vi "Servo Drive Test.vi"() -> ()   [LabVIEW 2020]
uses:
  <vilib>/MakerHub/LINX/LMH-LINX.lvlib
  LINX-PCA9685 PWM/LINX-PCA9685 PWM.lvclass
  LINX I2C/LINX I2C.lvclass
  <vilib>/MakerHub/LINX/Public/Utilities/Open Local.vi
panel:
  in  "PWM1":dbl(slide) scale=-100.0..100.0
  in  "PWM0":dbl(slide) scale=-100.0..100.0
  out "New Frequency (Hz)":dbl
  out "Initial Frequency (Hz)":dbl
  in  "stop":bool
  out "Error Out":errorcluster
  # "A simple example of driving two servo motors with a Raspberry Pi using the PCA9685 PWM driver chip.\n\nThe board provides 16 PWM channels for driving LEDs or Servos."
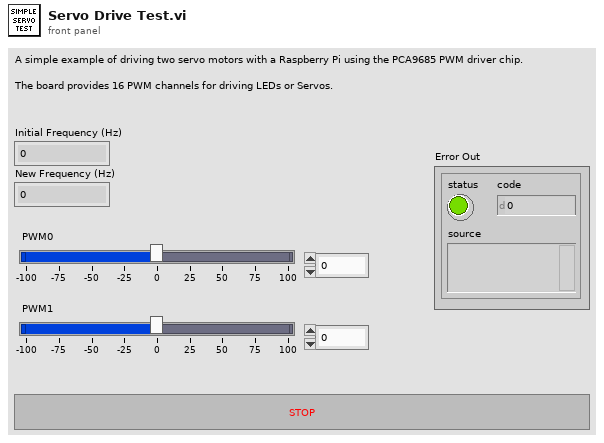
[diagram p1: front panel]
types:
  T1 = typedef "LMH-LINX.lvlib/LINX Ref.ctl" = cluster{"IO":T2, "Interface":T3, "LINX Device Config":T4}
  T2 = typedef "LMH-LINX.lvlib/Platform.ctl" = enum16{"Remote", "Local"}
  T3 = typedef "LMH-LINX.lvlib/Interface.ctl" = enum16{"Serial", "TCP"}
  T4 = typedef "LMH-LINX.lvlib/Device.lvlib/LINX Device Config.ctl" = cluster{"Interface":T3, "COM Port":refnum<visa-resource-name>, "TCP Configuration":T5, "Device Family":u8, "Device ID":u8, "Device Name":string, "TCP Ref":refnum<k5>, "Channels":T6}
  T5 = typedef "LMH-LINX.lvlib/Device.lvlib/TCP Config.ctl" = cluster{"IP Address":string, "Port":u16}
  T6 = typedef "LMH-LINX.lvlib/Channels.ctl" = cluster{"DI":u8[], "DO":u8[], "AI":u8[], "AO":u8[], "PWM":u8[], "QE":u8[], "UART":u8[], "I2C 2":u8[], "SPI":u8[], "CAN":u8[], "Servo":u8[], "AI Ref (V)":dbl, "AI Resolution (Bits)":u8, "AO Ref (V)":dbl, "AO Resolution (Bits)":u8}
  T7 = enum16{"LED/PWM00", "LED/PWM01", "LED/PWM02", "LED/PWM03", "LED/PWM04", "LED/PWM05", "LED/PWM06", "LED/PWM07", "LED/PWM08", "LED/PWM09", "LED/PWM10", "LED/PWM11", "LED/PWM12", "LED/PWM13", "LED/PWM14", "LED/PWM15"}[]
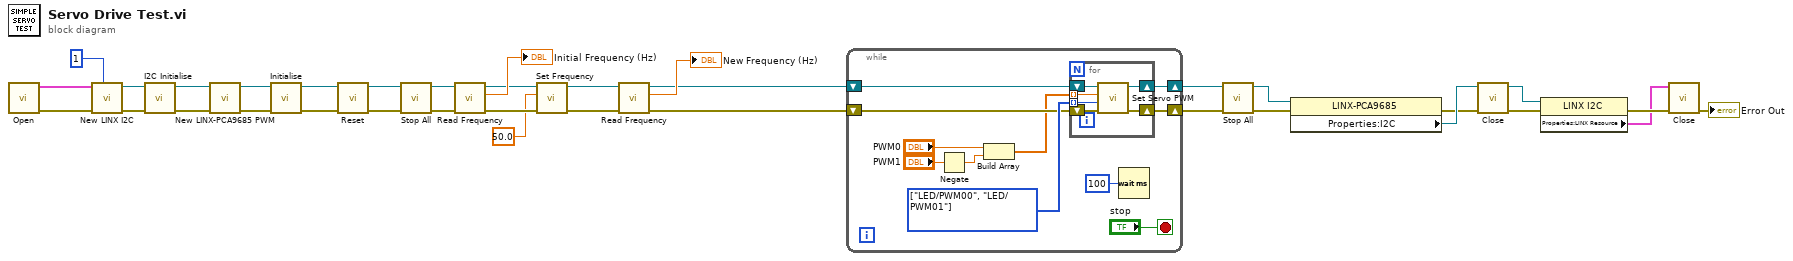
[diagram p0: block diagram]
diagram:
  n1 = call-poly <vilib>:"Open.vi"() -> ("Error Out"=w14:errorcluster, "LINX Resource"=w15:T1)  [unwired: 9 in, 1 out]
  n2 = call "New LINX I2C.vi"("LINX I2C Channel"=u8 1 ("I2C Channel"), "error in (no error)"=w14, "LINX Resource"=w15) -> ("error out"=w12:errorcluster, "LINX I2C out"=w11:refnum<class "LINX I2C.lvclass">)  [unwired: 7 in]
  n3 = call-dynamic "I2C Initialise.vi"("error in (no error)"=w12, "LINX I2C in"=w11) -> ("error out"=w4:errorcluster, "LINX I2C out"=w3:refnum<class "LINX I2C.lvclass">)  [unwired: 8 in]
  n4 = call "New LINX-PCA9685 PWM.vi"("error in (no error)"=w4, "I2C"=w3) -> ("error out"=w2:errorcluster, "LINX-PCA9865 PWM out"=w1:refnum<class "LINX-PCA9685 PWM.lvclass">)  [unwired: 8 in]
  n5 = call-dynamic "Initialise.vi"("error in (no error)"=w2, "PWM in"=w1) -> ("error out"=w19:errorcluster, "PWM out"=w20:refnum<class "LINX-PCA9685 PWM.lvclass">)  [unwired: 8 in]
  n6 = call-dynamic "Reset.vi"("error in (no error)"=w19, "PWM in"=w20) -> ("error out"=w18:errorcluster, "PWM out"=w17:refnum<class "LINX-PCA9685 PWM.lvclass">)  [unwired: 8 in]
  n7 = call-dynamic "Stop All.vi"("error in (no error)"=w18, "LINX-PCA9865 PWM in"=w17) -> ("error out"=w27:errorcluster, "LINX-PCA9865 PWM out"=w28:refnum<class "LINX-PCA9685 PWM.lvclass">)  [unwired: 8 in]
  n8 = call-dynamic "Read Frequency.vi"("error in (no error)"=w27, "PWM in"=w28) -> ("error out"=w33:errorcluster, "Frequency (Hz)"=→"Initial Frequency (Hz)":dbl, "PWM out"=w32:refnum<class "LINX-PCA9685 PWM.lvclass">)  [unwired: 7 in]
  n9 = call-dynamic "Set Frequency.vi"("error in (no error)"=w33, "Frequency (1000Hz)"=50.0, "PWM in"=w32) -> ("error out"=w31:errorcluster, "PWM out"=w30:refnum<class "LINX-PCA9685 PWM.lvclass">)  [unwired: 7 in]
  n10 = call-dynamic "Read Frequency.vi"("error in (no error)"=w31, "PWM in"=w30) -> ("error out"=w24:errorcluster, "Frequency (Hz)"=→"New Frequency (Hz)":dbl, "PWM out"=w25:refnum<class "LINX-PCA9685 PWM.lvclass">)  [unwired: 7 in]
  n11 = while {
    shift-right: [w43] -> w26
    shift-left: w24 -> [w40]
    shift-right: [w42] -> w23
    shift-left: w25 -> [w44]
    stop <- "stop" stop-if-true
    w41 = T7 [enum."LED/PWM00", enum."LED/PWM01"] items=["LED/PWM00", "LED/PWM01", "LED/PWM02", "LED/PWM03", "LED/PWM04", "LED/PWM05", "LED/PWM06", "LED/PWM07", "LED/PWM08", "LED/PWM09", "LED/PWM10", "LED/PWM11", "LED/PWM12", "LED/PWM13", "LED/PWM14", "LED/PWM15"] ("LEDn (PWM channel)")
    n12 = Negate(x="PWM1") -> (-x=w37:dbl)
    n13 = Build Array("PWM0", w37) -> (w36:dbl[])
    n14 = for {
      tunnel: w36 -> [w49] mode=indexing
      tunnel: w41 -> [w48] mode=indexing
      shift-right: [w50] -> w42
      shift-left: w44 -> [w52]
      shift-right: [w51] -> w43
      shift-left: w40 -> [w47]
      n15 = call "Set Servo PWM.vi"("error in (no error)"=w47, "LEDn (PWM channel)"=w48, "Servo Speed (-100 to 100%)"=w49, "LINX-PCA9865 PWM in"=w52) -> ("error out"=w51:errorcluster, "LINX-PCA9865 PWM out"=w50:refnum<class "LINX-PCA9685 PWM.lvclass">)  [unwired: 6 in]
    }
    n16 = Wait (ms)(milliseconds to wait=u32 100) -> ()  [unwired: 1 out]
  }
  n17 = call-dynamic "Stop All.vi"("error in (no error)"=w26, "LINX-PCA9865 PWM in"=w23) -> ("error out"=w21:errorcluster, "LINX-PCA9865 PWM out"=w22:refnum<class "LINX-PCA9685 PWM.lvclass">)  [unwired: 8 in]
  n18 = property class="LINX-PCA9685"(reference=w22, error in=w21) -> (error out=w9:errorcluster, "Properties:I2C"=w10:refnum<class "LINX I2C.lvclass">)  [unwired: 1 out]
  n19 = call-dynamic <vilib>:"Close.vi"("error in (no error)"=w9, "LINX I2C in"=w10) -> ("error out"=w8:errorcluster, "LINX I2C out"=w6:refnum<class "LINX I2C.lvclass">)  [unwired: 8 in]
  n20 = property class="LINX I2C"(reference=w6, error in=w8) -> (error out=w7:errorcluster, "Properties:LINX Resource"=w5:T1)  [unwired: 1 out]
  n21 = call <vilib>:"Close.vi"("Error In"=w7, "LINX Resource"=w5) -> ("Error Out"=→"Error Out":errorcluster)  [unwired: 9 in]
